vi "read analog.vi"(4 "Maximum Value":dbl=10.0 format="%0.2f", 6 "Minimum Value":dbl=-10.0 format="%0.2f", 8 "Physical Channel":refnum<k21>="Dev0/Ai1:0", 9 "Sample Rate":dbl=600.0 caption="Sample Rate (Hz)", 10 "clock source":i32(ring) items=["OnboardClock", "ExternalClock", "NoClock"], 11 "stop":bool) -> (3 "data":dbl[](array[numeric]))   [LabVIEW 2011]
uses:
  <vilib>/Utility/error.llb/DialogType.ctl
  <vilib>/ULx/Create Channel.llb/ULx Create Channel (AI-Voltage-Basic).vi
  <vilib>/ULx/Timing.llb/ULx Timing (Sample Clock).vi
  <vilib>/ULx/Read.llb/ULx Read (Analog 1D DBL NChan 1Samp).vi
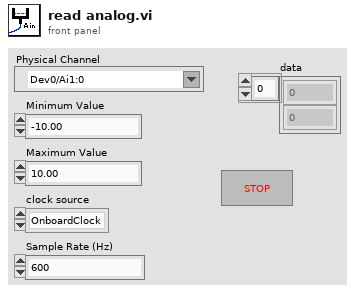
[diagram p1: front panel]
types:
  T1 = typedef "DialogType.ctl" = u16
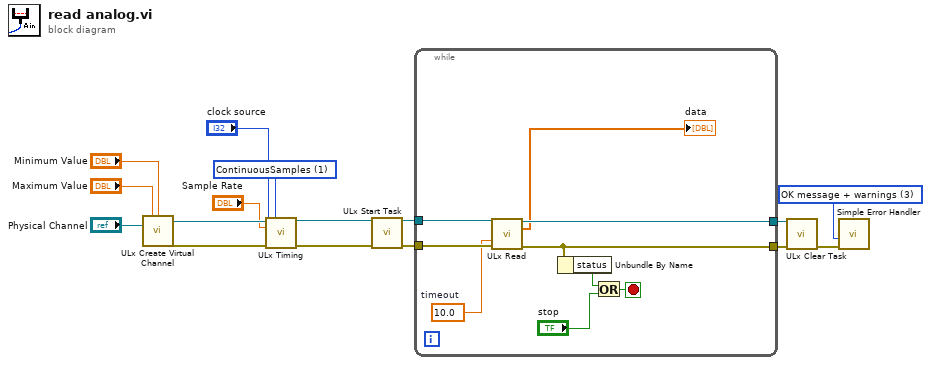
[diagram p0: block diagram]
diagram:
  w6 = 1 items=["FiniteSamples", "ContinuousSamples"] ("sample mode")
  w7 = T1 3 items=["no dialog", "OK message", "continue or stop message", "OK message + warnings", "continue/stop + warnings"] ("type of dialog (OK msg:1)")
  n1 = call-poly <vilib>:"ULx Create Virtual Channel.vi"("maximum value"="Maximum Value", "minimum value"="Minimum Value", "physical channels"="Physical Channel") -> ("task out"=w13:refnum<k24>, "error out"=w16:errorcluster)  [unwired: 11 in]
  n2 = call-poly <vilib>:"ULx Timing.vi"("task in"=w13, "sample mode"=w6, "rate"="Sample Rate", "clock source"="clock source", "error in"=w16) -> ("task out"=w10:refnum<k24>, "error out"=w9:errorcluster)  [unwired: 9 in]
  n3 = call <vilib>:"ULx Start Task.vi"("task in"=w10, "error in"=w9) -> ("task out"=w12:refnum<k24>, "error out"=w15:errorcluster)  [unwired: 12 in]
  n4 = while {
    tunnel: w15 -> [w25]
    tunnel: w12 -> [w24]
    tunnel: [w23] -> w11
    tunnel: [w22] -> w8
    stop <- w20 stop-if-true
    w18 = 10.0  # timeout
    n5 = call-poly <vilib>:"ULx Read.vi"("task in"=w24, "timeout"=w18, "error in"=w25) -> ("task out"=w23:refnum<k24>, "data"=→"data":dbl[], "error out"=w22:errorcluster)  [unwired: 10 in]
    n6 = Unbundle By Name(w22) -> ("status"=w21:bool)
    n7 = Or(x=w21, y="stop") -> (x .or. y?=w20:bool)
  }
  n8 = call <vilib>:"ULx Clear Task.vi"("task in"=w11, "error in"=w8) -> ("error out"=w14:errorcluster)  [unwired: 13 in]
  n9 = call <vilib>:"Simple Error Handler.vi"("type of dialog (OK msg:1)"=w7, "error in (no error)"=w14) -> ()  [unwired: 3 in, 5 out]
